vi "Stop.vi"(8 "error in (no error)":errorcluster, 11 "Motor in":refnum<class "Motor.lvclass">) -> (0 "error out":errorcluster, 3 "Motor out":refnum<class "Motor.lvclass">)   [LabVIEW 2019, in "Motor.lvclass"]
uses:
  Motor.lvclass
  Motor.lvclass/Motor.ctl
  Motor Serial class/Serial.lvclass
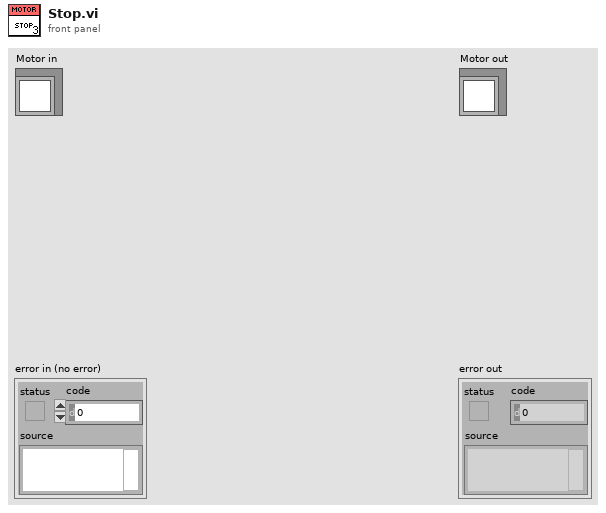
[diagram p1: front panel]
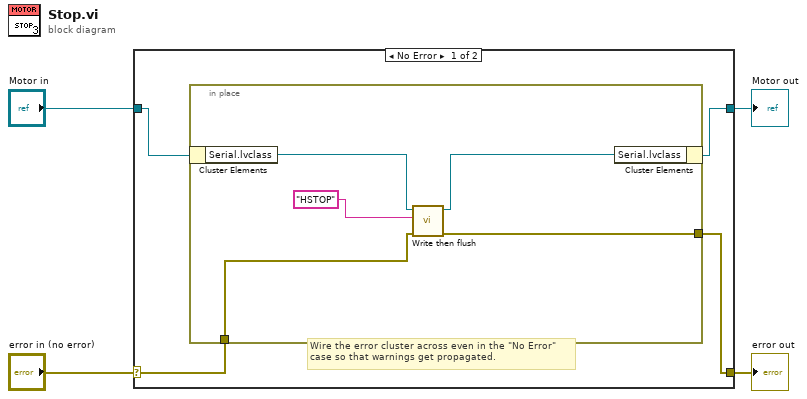
[diagram p0: block diagram]
diagram:
  n1 = case shown="No Error" "error in (no error)" {
    selector: "error in (no error)" -> [w5 w15]
    tunnel: [w6 w15] -> w3
    tunnel: [w7 w14] -> w1
    tunnel: "Motor in" -> [w8 w14]
    frame No Error {
      # "Wire the error cluster across even in the \"No Error\"\ncase so that warnings get propagated."
      n2 = in-place {
        in-place-border: [w11] -> w6
        in-place-border: w5 -> [w10]
        n3 = in-place-cluster #1(w8) -> ("Serial.lvclass"=w13:refnum<class "Serial.lvclass">)
        n4 = call "Write then flush.vi"("error in (no error)"=w10, "TX Data"="HSTOP" ("string"), "Motor_Serial in"=w13) -> ("error out"=w11:errorcluster, "Motor_Serial out"=w12:refnum<class "Serial.lvclass">)  [unwired: 7 in]
        n5 = in-place-cluster #1("Serial.lvclass"=w12) -> (w7:refnum<class "Motor.lvclass">)
      }
    }
    frame Error {
    }
  }
  "error out" <- w3
  "Motor out" <- w1
